vi "BMPtoPNG.vi"(8 "error in":errorcluster, 11 "image path in (.bmp)":path) -> (0 "error out":errorcluster, 3 "image path out (.png)":path)   [LabVIEW 2019]
panel:
  out "File Data Type out":i32
  # "BMPTOPNG"
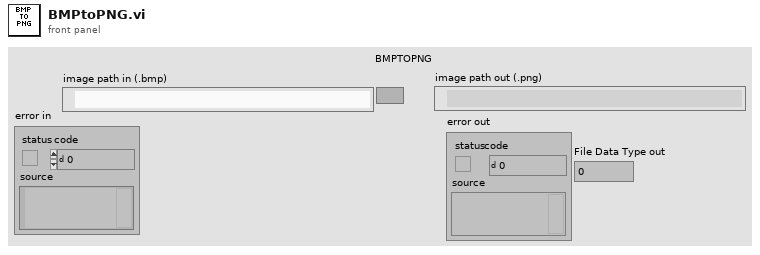
[diagram p1: front panel]
types:
  T1 = typedef "Image Type" = u32
  T2 = typedef "IMAQ Image.ctl" = refnum<image>
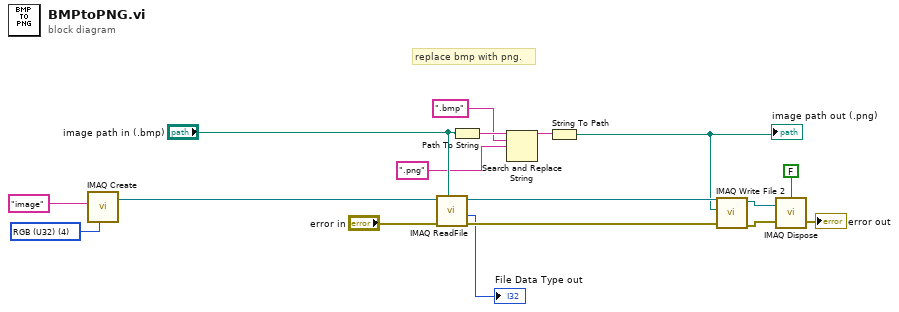
[diagram p0: block diagram]
diagram:
  w14 = T1 4 items=["Grayscale (U8)", "Grayscale (I16)", "Grayscale (SGL)", "Complex (CSG)", "RGB (U32)", "HSL (U32)", "RGB (U64)", "Grayscale (U16)"] ("Image Type")
  # "replace bmp with png."
  n1 = call "IMAQ Create"("Image Name"="image", "Image Type"=w14) -> ("New Image"=w13:T2)  [unwired: 3 in, 1 out]
  n2 = call "IMAQ ReadFile"("File Path"="image path in (.bmp)", "error in (no error)"="error in", "Image"=w13) -> ("error out"=w16:errorcluster, "File Data Type out"=→"File Data Type out":i32, "Image Out"=w17:T2)  [unwired: 4 in, 2 out]
  n3 = Path To String(path="image path in (.bmp)") -> (string=w5:string)
  n4 = Search and Replace String(input string=w5, search string=".bmp", replace string=".png" ("replace string (\"\")")) -> (result string=w1:string)  [unwired: 5 in, 3 out]
  n5 = String To Path(string=w1) -> (path=w3:path)
  "image path out (.png)" <- w3
  n6 = call-poly "IMAQ Write File 2"("error in (no error)"=w16, "File Path"=w3, "Image"=w17) -> ("error out"=w11:errorcluster, "Image Out (duplicate)"=w12:T2)  [unwired: 7 in]
  n7 = call "IMAQ Dispose"("All Images? (No)"=FALSE, "Image"=w12, "error in (no error)"=w11) -> ("error out"=→"error out":errorcluster)  [unwired: 3 in]
